vi "NI 9215 Getting Started (FPGA).vi"() -> ()   [LabVIEW 2018]
uses:
  <vilib>/rvi/Emulation/niFpgaGetClockAttributes.vi
  <vilib>/rvi/Emulation/niFpgaSctlEmulationGetInTimedLoop.vi
  <vilib>/rvi/Emulation/niFpgaEmulationReportErrorSimple.vi
  Instance           1 31Saved   NI 9203 Basic IO (FPGA) .vi
  <vilib>/rvi/eio/common/nirviEmuTemplateMethod_errors.vi
  <vilib>/rvi/interface/RandomDataEmulation/niFpgaRandomDataHandleErrors.vi
  <vilib>/rvi/Emulation/niFpgaCriticalErrorInLSC.vi
  <vilib>/eio/EIONode/EIONode.xnode
  <vilib>/rvi/DataTransferAndStorage/Container/XNode/niFpgaContainer.xnode
  <vilib>/rvi/interface/RandomDataEmulation/nirviRandomDataFpgaReadWriteTemplate.vi
panel:
  out "FPGA Error Out":errorcluster
  in  "Stop":bool
  in  "Loop Rate (uS)":u32
  out "Data FIFO Full":bool
  # "Overview: Demonstrates how to acquire and scale the data from the NI 9215. \nRequirements: LabVIEW Full Development System, LV FPGA, and NI RIO\nInstructions: \n1. Run NI 9201 Getting Started (Host)"
  # "Input Parameters"
  # "Error Cluster"
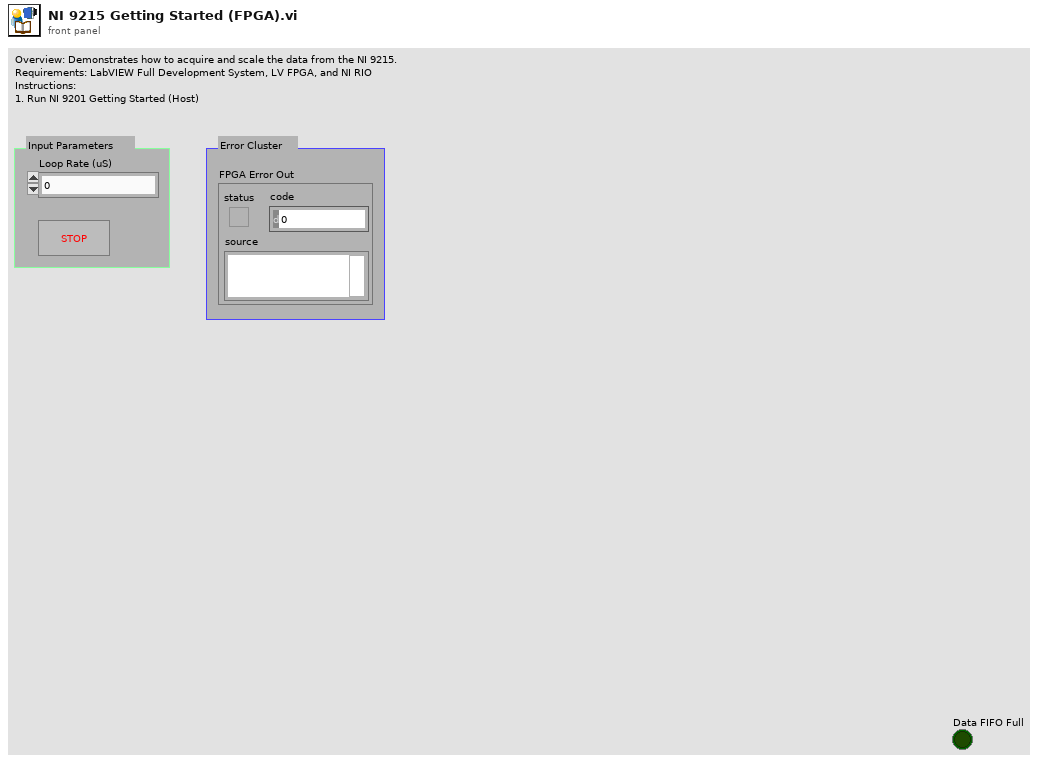
[diagram p1: front panel]
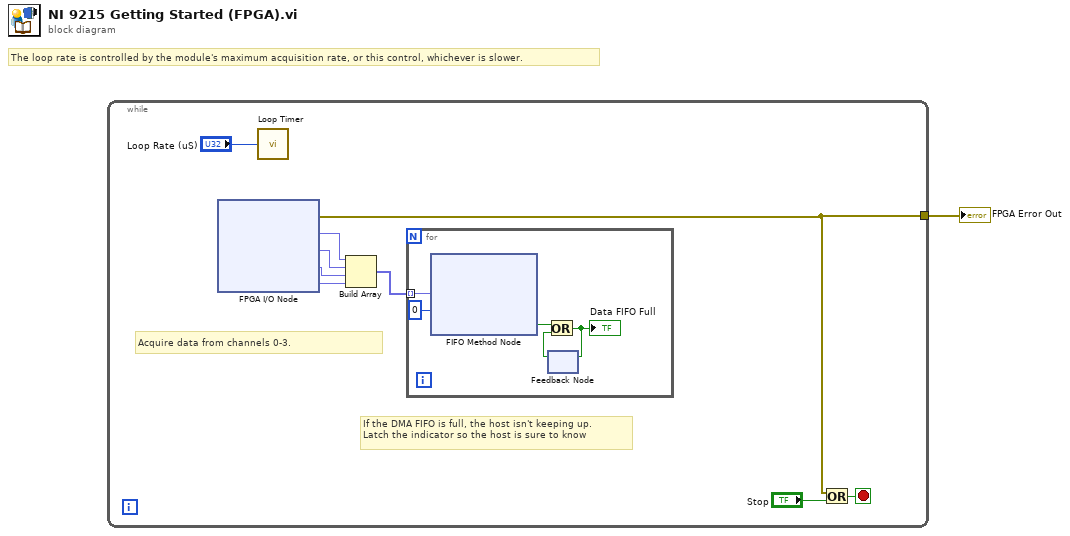
[diagram p0: block diagram]
diagram:
  # "The loop rate is controlled by the module's maximum acquisition rate, or this control, whichever is slower."
  n1 = while {
    tunnel: [w2] -> w1
    stop <- w3 stop-if-true
    # "Acquire data from channels 0-3."
    # "If the DMA FIFO is full, the host isn't keeping up. \nLatch the indicator so the host is sure to know"
    n2 = xnode "FPGA I/O Node"() -> ("error out"=w2:errorcluster, "Mod1/AI0"=w7:fxp<+/-,20,5>, "Mod1/AI1"=w6:fxp<+/-,20,5>, "Mod1/AI2"=w5:fxp<+/-,20,5>, "Mod1/AI3"=w4:fxp<+/-,20,5>)  [unwired: 5 in, 4 out]
    n3 = call "Loop Timer"("Count(uSec)"="Loop Rate (uS)") -> ()  [unwired: 1 out]
    n4 = Build Array(w7, w6, w5, w4) -> (w8:fxp<+/-,20,5>[])
    n5 = for {
      tunnel: w8 -> [w15] mode=indexing
      n6 = xnode ("FIFO Method Node")("Element"=w15, "Timeout"=0) -> ("Timed Out?"=w11:bool)  [unwired: 1 in, 1 out]
      n7 = feedback #1() -> (w13:bool)  [unwired: 1 out]
      n8 = Or(x=w11, y=w13) -> (x .or. y?=w12:bool)
      "Data FIFO Full" <- w12
      n9 = feedback-in #1(w12) -> ()
    }
    n10 = Or(x=w2, y="Stop") -> (x .or. y?=w3:bool)
  }
  "FPGA Error Out" <- w1
